vi "Control Panel(WIP).vi"(8 "error in (no error)":errorcluster, 11 "Lockin SR830 in":refnum<class "Lockin SR830.lvclass">) -> (0 "error out":errorcluster, 3 "Lockin SR830 out":refnum<class "Lockin SR830.lvclass">)   [LabVIEW 2017, in "Lockin SR830.lvclass"]
uses:
  Lockin SR830.lvclass
  Lockin SR830.lvclass/Lockin SR830.ctl
  sr830/SR830.lvlib
panel:
  out "?":enum32{"Page 1", "Page 2"}(tab)
  out "Channel 2 Display":dbl
  out "Channel 1 Display":dbl
  out "Ref Freq":dbl[unit]
  in  "Ch 1 Option":T1(ring)
  in  "Ch 2 Option":T2(ring)
  out "Channel 1 display":dbl
  out "Ref freq":dbl[unit]
  in  "Ch 1 option":T1(ring)
  out "Phase":dbl format="%#_13g"
  in  "autophase":bool
  out "External ref":bool=TRUE
  in  "External ref?":bool=TRUE
  in  "Read":bool
  in  "Copy actual to set":bool
  in  "Populate fields with member data":bool
  in  "endprgm":bool
  in  "set":bool
  out "sensdisp":T3(ring) caption="Sensitivity"
  out "tcdisp":T4(ring) caption="Time Const."
  in  "sens":T3(ring) caption="Sensitivity"
  in  "tc":T4(ring) caption="Time Const."
  # "Lock-in Detector Front Panel"
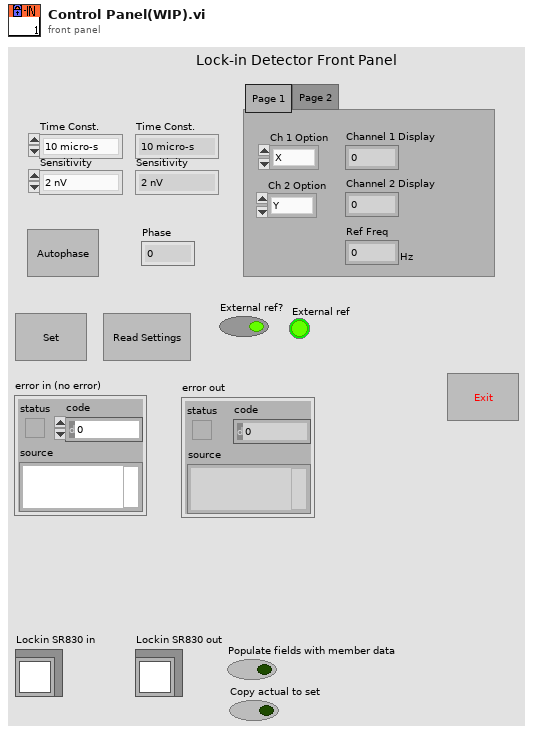
[diagram p1: front panel]
types:
  T1 = enum16{"X", "R", "X Noise", "Aux in 1", "Aux in 2"}
  T2 = enum16{"Y", "Theta", "Y Noise", "Aux in 3", "Aux in 4"}
  T3 = enum16{"2 nV", "5 nV", "10 nV", "20 nV", "50 nV", "100 nV", "200 nV", "500 nV", "1 microV", "2 microV", "5 microV", "10 microV", "20 microV", "50  microV", "100  microV", "200  microV", "500  microV", "1 mV", "2 mV", "5 mV", "10 mV", "20 mV", "50 mV", "100 mV", "200  mV", "500 mV", "1 V"}
  T4 = enum16{"10 micro-s", "30 micro-s", "100 micro-s", "300 micro-s", "1 ms", "3 ms", "10 ms", "30 ms", "100 ms", "300 ms", "1 s", "3 s", "10 s", "30 s", "100 s", "300 s", "1000 s", "30000 s", "10 ks", "30 ks"}
  T5 = typedef "Lockin SR830.lvclass/Sensitivity.ctl" = u16
  T6 = typedef "SR830.lvlib/Tau.ctl" = u16
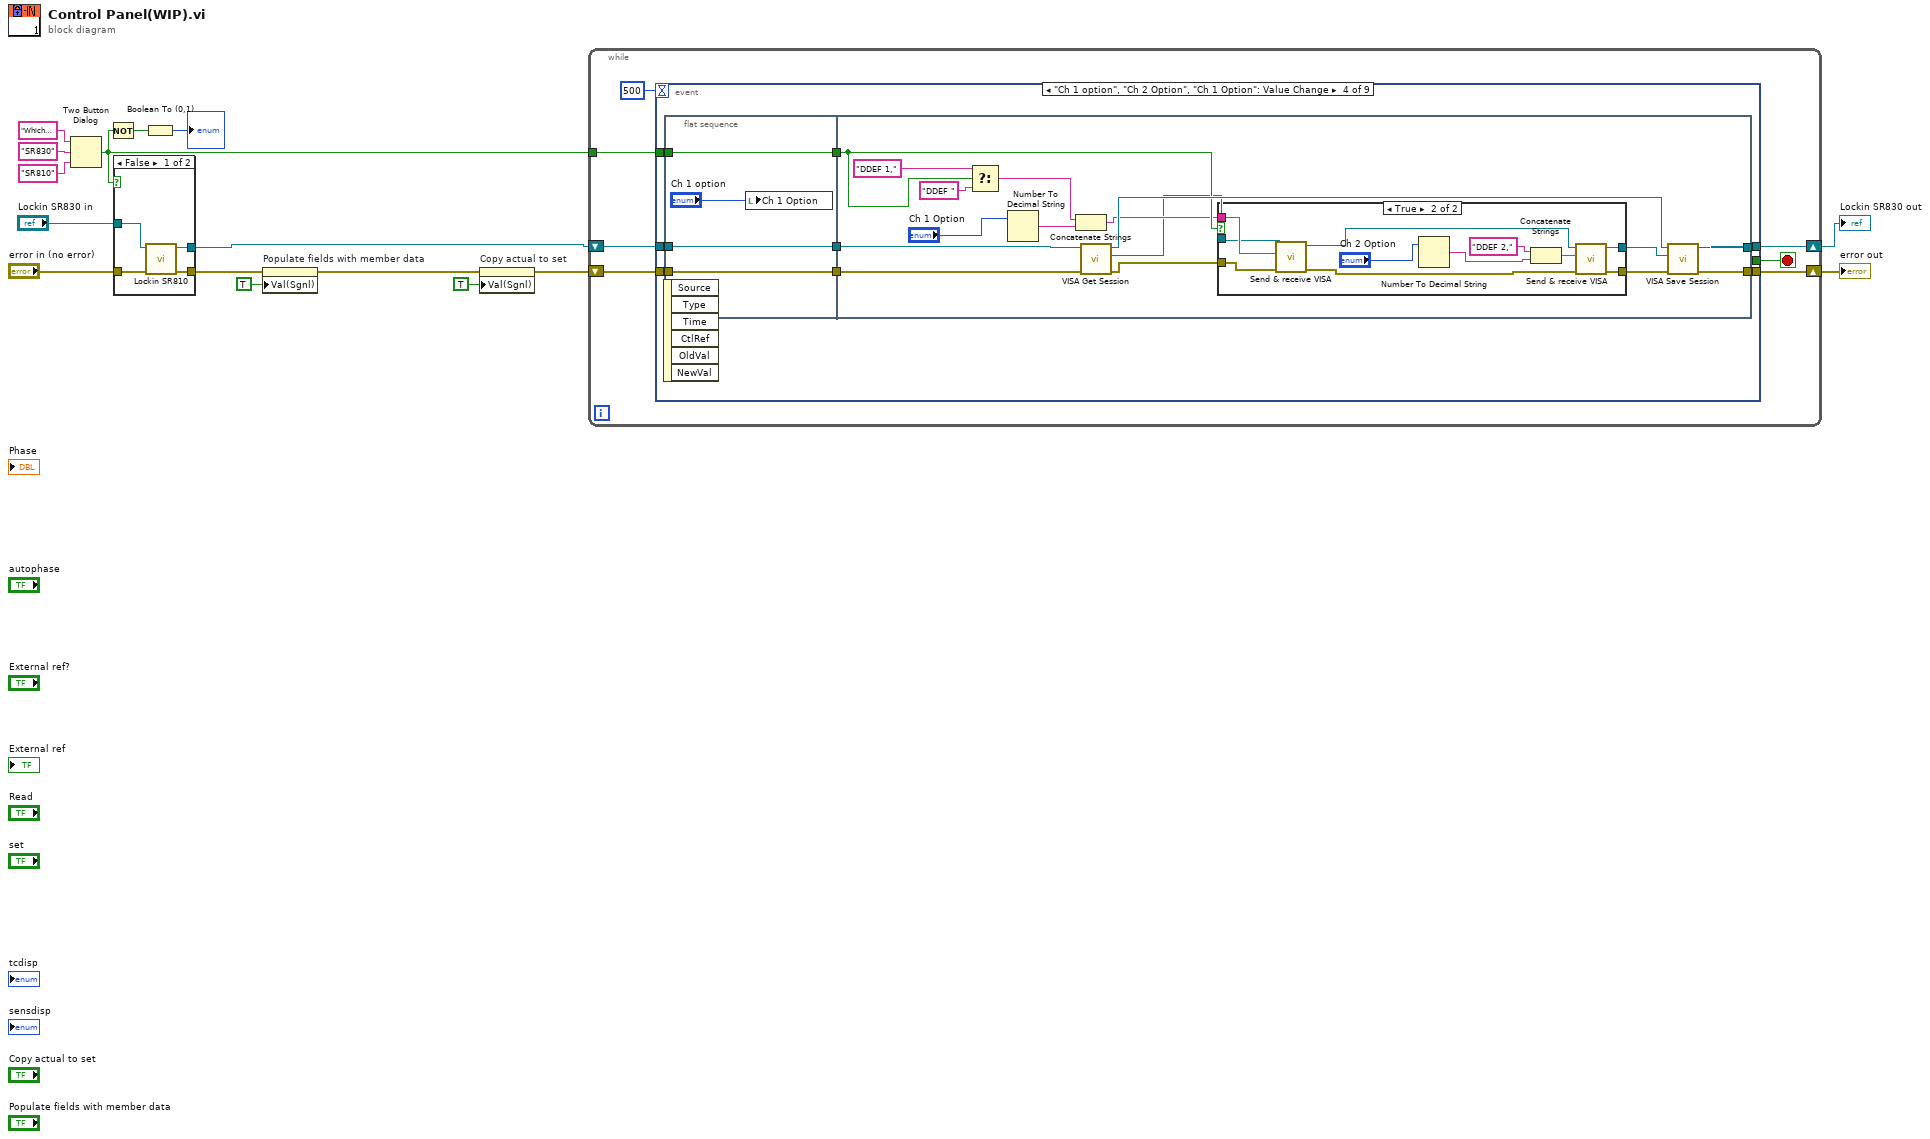
[diagram p0: block diagram]
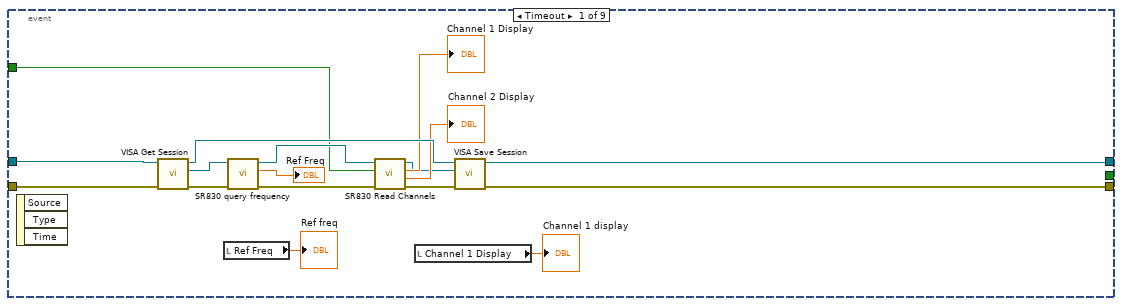
[diagram p2: hidden frame]
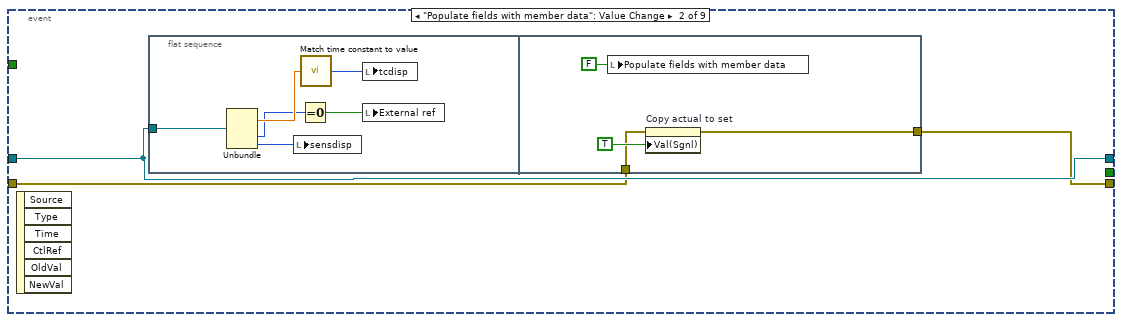
[diagram p3: hidden frame]
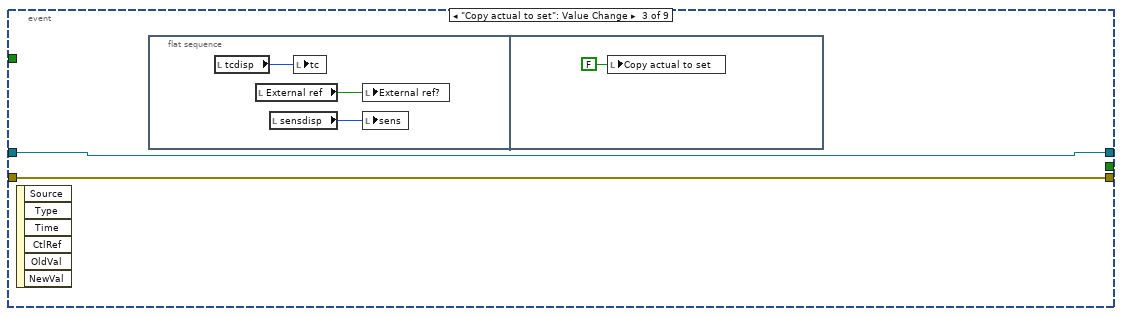
[diagram p4: hidden frame]
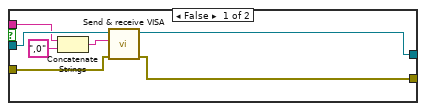
[diagram p5: hidden frame]
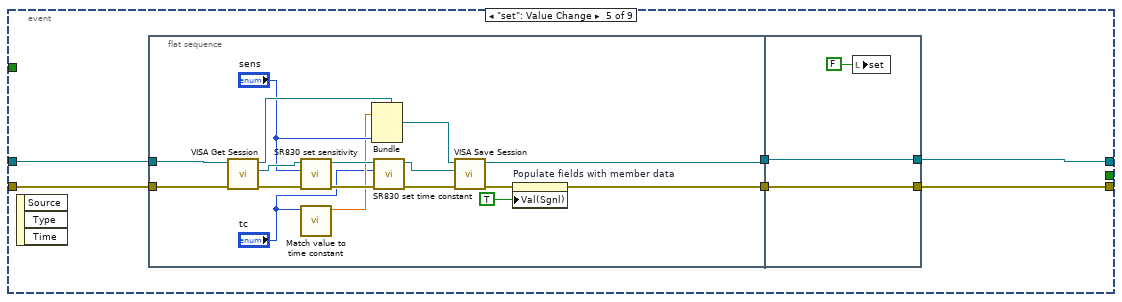
[diagram p6: hidden frame]
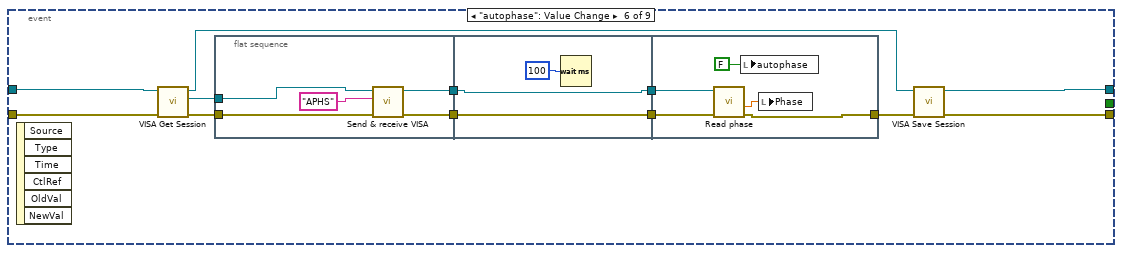
[diagram p7: hidden frame]
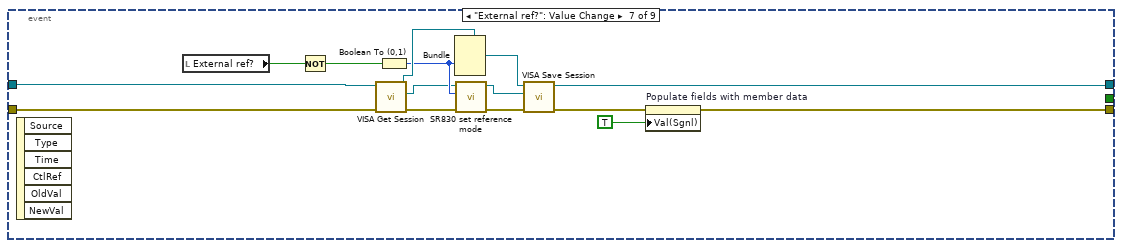
[diagram p8: hidden frame]
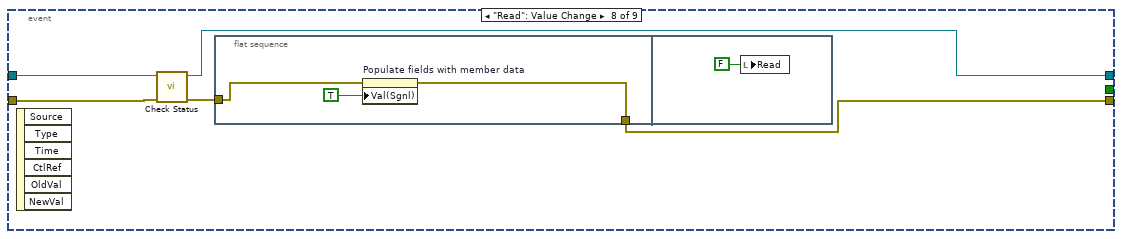
[diagram p9: hidden frame]
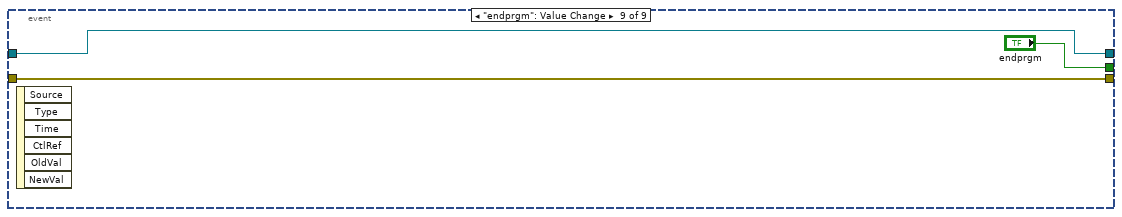
[diagram p10: hidden frame]
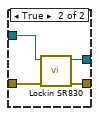
[diagram p11: hidden frame]
diagram:
  n1 = Two Button Dialog(message="Which model Lock-In are you using?", 1:"SR810" ("F button name (\"Cancel\")"), 2:"SR830" ("T button name (\"OK\")")) -> (T button?=w1:bool)
  n2 = Not(x=w1) -> (.not. x?=w3:bool)
  n3 = case shown="False" w1 {
    tunnel: "Lockin SR830 in" -> [w20 w24]
    tunnel: "error in (no error)" -> [w18 w23]
    tunnel: [w17 w22] -> w8
    tunnel: [w19 w21] -> w13
    frame False {
      n4 = call "Lockin SR810.vi"("error in (no error)"=w18, "Lockin SR830 in"=w20) -> ("error out"=w17:errorcluster, "Lockin SR830 out"=w19:refnum<class "Lockin SR830.lvclass">)  [unwired: 8 in]
    }
    frame True {
      n5 = call "Lockin SR830.vi"("error in (no error)"=w23, "Lockin SR830 in"=w24) -> ("error out"=w22:errorcluster, "Lockin SR830 out"=w21:refnum<class "Lockin SR830.lvclass">)  [unwired: 8 in]
    }
  }
  n6 = Boolean To (0,1)(Boolean=w3) -> (0, 1=→"?":i16)
  n7 = property on="Populate fields with member data" class="Bool (strict)"(error in=w8, "Val(Sgnl)"=TRUE) -> (error out=w7:errorcluster)  [unwired: 1 in, 1 out]
  n8 = property on="Copy actual to set" class="Bool (strict)"(error in=w7, "Val(Sgnl)"=TRUE) -> (error out=w6:errorcluster)  [unwired: 1 in, 1 out]
  n9 = while {
    shift-right: [w27] -> w14
    shift-left: w13 -> [w28]
    shift-right: [w29] -> w9
    shift-left: w6 -> [w30]
    tunnel: w1 -> [w25]
    stop <- w31 stop-if-true
    n10 = event shown="[3] \"Ch 1 option\", \"Ch 2 Option\", \"Ch 1 Option\": Value Change" {
      selector: _ -> [_ _ _ _ _ _ _ _ _]
      dyn-events: _ -> [_ _ _ _ _ _ _ _ _]
      timeout: 500 -> [_ _ _ _ _ _ _ _ _]
      tunnel: [_ _ _ _ _ _ _ _ "endprgm"] -> w31
      tunnel: w28 -> [w48 w51 w63 w75 w119 w151 w169 w184 w189]
      tunnel: w30 -> [w44 w50 w62 w74 w118 w148 w167 w183 w190]
      tunnel: [w35 w49 w62 w73 w117 w140 w168 w181 w190] -> w29
      tunnel: [w46 w51 w63 w72 w116 w149 w170 w180 w189] -> w27
      tunnel: w25 -> [w34 _ _ w71 _ _ _ _ _]
      event Timeout {
        n11 = event-data() -> ()  [unwired: 1 in, 3 out]
        n12 = call-dynamic "VISA Get Session.vi"("error in (no error)"=w44, "Instrument.lvclass in"=w48) -> ("error out"=w43:errorcluster, "VISA Resource Name"=w45:refnum<visa-resource-name>, "Instrument.lvclass out"=w47:refnum<class "Lockin SR830.lvclass">)  [unwired: 7 out]
        n13 = local read "Ref Freq"() -> (→"Ref freq":dbl[unit])
        n14 = call "SR830 query frequency.vi"("error in (no error)"=w43, "VISA resource name"=w45) -> ("error out"=w40:errorcluster, "frequency"=→"Ref Freq":dbl[unit], "VISA resource name out"=w41:refnum<visa-resource-name>)  [unwired: 7 in]
        n15 = call "SR830 Read Channels.vi"("error in (no error)"=w40, "830?"=w34, "VISA Resource Name"=w41) -> ("error out"=w36:errorcluster, "output2"=→"Channel 2 Display":dbl, "output1"=→"Channel 1 Display":dbl, "VISA resource name out"=w37:refnum<visa-resource-name>)  [unwired: 5 in]
        n16 = local read "Channel 1 Display"() -> (→"Channel 1 display":dbl)
        n17 = call-dynamic "VISA Save Session.vi"("error in (no error)"=w36, "VISA Resource Name"=w37, "Instrument.lvclass in"=w47) -> ("error out"=w35:errorcluster, "Instrument.lvclass out"=w46:refnum<class "Lockin SR830.lvclass">)  [unwired: 7 out]
      }
      event "Populate fields with member data": Value Change {
        n18 = event-data() -> ()  [unwired: 1 in, 6 out]
        n19 = flat-sequence {
          tunnel: w51 -> [w56]
          tunnel: [w58] -> w49
          tunnel: w50 -> [w59]
          frame #0 {
            n20 = Unbundle(w56) -> (w55:dbl[unit], w52:enum16{"external", "internal"}, w57:T5)  [unwired: 2 out]
            n21 = local write "sensdisp"(w57) -> ()
            n22 = Equal To 0?(x=w52) -> (x = 0?=w53:bool)
            n23 = call "Match time constant to value.vi"("Time constant"=w55) -> ("Tau"=w54:T6)
            n24 = local write "tcdisp"(w54) -> ()
            n25 = local write "External ref"(w53) -> ()
          }
          frame #1 {
            n26 = local write "Populate fields with member data"(FALSE) -> ()
            n27 = property on="Copy actual to set" class="Bool (strict)"(error in=w59, "Val(Sgnl)"=TRUE) -> (error out=w58:errorcluster)  [unwired: 1 in, 1 out]
          }
        }
      }
      event "Copy actual to set": Value Change {
        n28 = event-data() -> ()  [unwired: 1 in, 6 out]
        n29 = flat-sequence {
          frame #0 {
            n30 = local read "tcdisp"() -> (w66:T4)
            n31 = local read "External ref"() -> (w64:bool)
            n32 = local read "sensdisp"() -> (w65:T3)
            n33 = local write "tc"(w66) -> ()
            n34 = local write "External ref?"(w64) -> ()
            n35 = local write "sens"(w65) -> ()
          }
          frame #1 {
            n36 = local write "Copy actual to set"(FALSE) -> ()
          }
        }
      }
      event "Ch 1 option", "Ch 2 Option", "Ch 1 Option": Value Change {
        n37 = event-data() -> ()  [unwired: 1 in, 6 out]
        n38 = flat-sequence {
          tunnel: w71 -> [w77]
          tunnel: w74 -> [w78]
          tunnel: w75 -> [w79]
          tunnel: [w79] -> w70
          tunnel: [w78] -> w69
          tunnel: [w77] -> w68
          tunnel: [w92] -> w73
          tunnel: [w91] -> w72
          tunnel: w70 -> [w95]
          tunnel: w69 -> [w93]
          tunnel: w68 -> [w86]
          frame #0 {
            n39 = local write "Ch 1 Option"("Ch 1 option") -> ()
          }
          frame #1 {
            n40 = Select(t="DDEF 1," ("write buffer"), s=w86, f="DDEF " ("write buffer")) -> (s? t:f=w83:string)
            n41 = Number To Decimal String(number="Ch 1 Option") -> (decimal integer string=w87:string)  [unwired: 1 in]
            n42 = Concatenate Strings(w83, w87) -> (w81:string)
            n43 = call-dynamic "VISA Get Session.vi"("error in (no error)"=w93, "Instrument.lvclass in"=w95) -> ("error out"=w82:errorcluster, "VISA Resource Name"=w80:refnum<visa-resource-name>, "Instrument.lvclass out"=w94:refnum<class "Lockin SR830.lvclass">)  [unwired: 7 out]
            n44 = case shown="True" w86 {
              tunnel: [w96 w113] -> w90
              tunnel: [w97 w112] -> w89
              tunnel: w82 -> [w98 w107]
              tunnel: w81 -> [w101 w106]
              tunnel: w80 -> [w102 w105]
              frame False {
                n45 = Concatenate Strings(w101, ",0" ("string")) -> (w99:string)
                n46 = call "Send & receive VISA.vi"("error in (no error)"=w98, "write buffer"=w99, "VISA resource name"=w102) -> ("error out"=w97:errorcluster, "VISA resource name out"=w96:refnum<visa-resource-name>)  [unwired: 5 in, 2 out]
              }
              frame True {
                n47 = call "Send & receive VISA.vi"("error in (no error)"=w107, "write buffer"=w106, "VISA resource name"=w105) -> ("error out"=w104:errorcluster, "VISA resource name out"=w103:refnum<visa-resource-name>)  [unwired: 5 in, 2 out]
                n48 = Number To Decimal String(number="Ch 2 Option") -> (decimal integer string=w111:string)  [unwired: 1 in]
                n49 = Concatenate Strings("DDEF 2," ("write buffer"), w111) -> (w109:string)
                n50 = call "Send & receive VISA.vi"("error in (no error)"=w104, "write buffer"=w109, "VISA resource name"=w103) -> ("error out"=w112:errorcluster, "VISA resource name out"=w113:refnum<visa-resource-name>)  [unwired: 5 in, 2 out]
              }
            }
            n51 = call-dynamic "VISA Save Session.vi"("error in (no error)"=w89, "VISA Resource Name"=w90, "Instrument.lvclass in"=w94) -> ("error out"=w92:errorcluster, "Instrument.lvclass out"=w91:refnum<class "Lockin SR830.lvclass">)  [unwired: 7 out]
          }
        }
      }
      event "set": Value Change {
        n52 = event-data() -> ()  [unwired: 1 in, 3 out]
        n53 = flat-sequence {
          tunnel: w119 -> [w136]
          tunnel: w118 -> [w134]
          tunnel: [w127] -> w115
          tunnel: [w130] -> w114
          tunnel: [w138] -> w116
          tunnel: [w139] -> w117
          tunnel: w115 -> [w139]
          tunnel: w114 -> [w138]
          frame #0 {
            n54 = call-dynamic "VISA Get Session.vi"("error in (no error)"=w134, "Instrument.lvclass in"=w136) -> ("error out"=w133:errorcluster, "VISA Resource Name"=w135:refnum<visa-resource-name>, "Instrument.lvclass out"=w126:refnum<class "Lockin SR830.lvclass">)  [unwired: 7 out]
            n55 = call "SR830 set sensitivity.vi"("error in (no error)"=w133, "Sensitivity"="sens", "VISA resource name"=w135) -> ("error out"=w131:errorcluster, "VISA resource name out"=w132:refnum<visa-resource-name>)  [unwired: 7 in]
            n56 = call "Match value to time constant.vi"("Tau"="tc") -> ("time constant"=w123:dbl[unit])  [unwired: 10 in]
            n57 = Bundle(cluster=w126, w123, "sens") -> (w124:refnum<class "Lockin SR830.lvclass">)  [unwired: 3 in]
            n58 = call "SR830 set time constant.vi"("error in (no error)"=w131, "Tau"="tc", "VISA resource name"=w132) -> ("error out"=w121:errorcluster, "VISA resource name out"=w120:refnum<visa-resource-name>)  [unwired: 7 in]
            n59 = call-dynamic "VISA Save Session.vi"("error in (no error)"=w121, "VISA Resource Name"=w120, "Instrument.lvclass in"=w124) -> ("error out"=w128:errorcluster, "Instrument.lvclass out"=w130:refnum<class "Lockin SR830.lvclass">)  [unwired: 7 out]
            n60 = property on="Populate fields with member data" class="Bool (strict)"(error in=w128, "Val(Sgnl)"=TRUE) -> (error out=w127:errorcluster)  [unwired: 1 in, 1 out]
          }
          frame #1 {
            n61 = local write "set"(FALSE) -> ()
          }
        }
      }
      event "autophase": Value Change {
        n62 = event-data() -> ()  [unwired: 1 in, 6 out]
        n63 = call-dynamic "VISA Get Session.vi"("error in (no error)"=w148, "Instrument.lvclass in"=w151) -> ("error out"=w146:errorcluster, "VISA Resource Name"=w147:refnum<visa-resource-name>, "Instrument.lvclass out"=w150:refnum<class "Lockin SR830.lvclass">)  [unwired: 7 out]
        n64 = flat-sequence {
          tunnel: w147 -> [w156]
          tunnel: w146 -> [w155]
          tunnel: [w153] -> w144
          tunnel: [w152] -> w142
          tunnel: [w158] -> w145
          tunnel: w144 -> [w158]
          tunnel: [w157] -> w143
          tunnel: w142 -> [w157]
          tunnel: w145 -> [w164]
          tunnel: w143 -> [w163]
          tunnel: [w161] -> w141
          frame #0 {
            n65 = call "Send & receive VISA.vi"("error in (no error)"=w155, "write buffer"="APHS", "VISA resource name"=w156) -> ("error out"=w152:errorcluster, "VISA resource name out"=w153:refnum<visa-resource-name>)  [unwired: 5 in, 2 out]
          }
          frame #1 {
            n66 = Wait (ms)(milliseconds to wait=u32 100) -> ()  [unwired: 1 out]
          }
          frame #2 {
            n67 = call "Read phase.vi"("error in (no error)"=w163, "VISA resource name"=w164) -> ("error out"=w161:errorcluster, "phase"=w162:dbl)  [unwired: 7 in, 1 out]
            n68 = local write "autophase"(FALSE) -> ()
            n69 = local write "Phase"(w162) -> ()
          }
        }
        n70 = call-dynamic "VISA Save Session.vi"("error in (no error)"=w141, "Instrument.lvclass in"=w150) -> ("error out"=w140:errorcluster, "Instrument.lvclass out"=w149:refnum<class "Lockin SR830.lvclass">)  [unwired: 1 in, 7 out]
      }
      event "External ref?": Value Change {
        n71 = event-data() -> ()  [unwired: 1 in, 6 out]
        n72 = local read "External ref?"() -> (w172:bool)
        n73 = Not(x=w172) -> (.not. x?=w173:bool)
        n74 = call-dynamic "VISA Get Session.vi"("error in (no error)"=w167, "Instrument.lvclass in"=w169) -> ("error out"=w166:errorcluster, "VISA Resource Name"=w165:refnum<visa-resource-name>, "Instrument.lvclass out"=w177:refnum<class "Lockin SR830.lvclass">)  [unwired: 7 out]
        n75 = Boolean To (0,1)(Boolean=w173) -> (0, 1=w171:i16)
        n76 = Bundle(cluster=w177, w171) -> (w176:refnum<class "Lockin SR830.lvclass">)  [unwired: 4 in]
        n77 = call "SR830 set reference mode.vi"("error in (no error)"=w166, "reference mode"=w171, "VISA resource name"=w165) -> ("error out"=w175:errorcluster, "VISA resource name out"=w174:refnum<visa-resource-name>)  [unwired: 7 in]
        n78 = call-dynamic "VISA Save Session.vi"("error in (no error)"=w175, "VISA Resource Name"=w174, "Instrument.lvclass in"=w176) -> ("error out"=w178:errorcluster, "Instrument.lvclass out"=w170:refnum<class "Lockin SR830.lvclass">)  [unwired: 7 out]
        n79 = property on="Populate fields with member data" class="Bool (strict)"(error in=w178, "Val(Sgnl)"=TRUE) -> (error out=w168:errorcluster)  [unwired: 1 in, 1 out]
      }
      event "Read": Value Change {
        n80 = event-data() -> ()  [unwired: 1 in, 6 out]
        n81 = call-dynamic "Check Status.vi"("error in (no error)"=w183, "Lockin SR830 in"=w184) -> ("error out"=w182:errorcluster, "Lockin SR830 out"=w180:refnum<class "Lockin SR830.lvclass">)  [unwired: 6 in, 2 out]
        n82 = flat-sequence {
          tunnel: w182 -> [w186]
          tunnel: [w185] -> w181
          frame #0 {
            n83 = property on="Populate fields with member data" class="Bool (strict)"(error in=w186, "Val(Sgnl)"=TRUE) -> (error out=w185:errorcluster)  [unwired: 1 in, 1 out]
          }
          frame #1 {
            n84 = local write "Read"(FALSE) -> ()
          }
        }
      }
      event "endprgm": Value Change {
        n85 = event-data() -> ()  [unwired: 1 in, 6 out]
      }
    }
  }
  "error out" <- w9
  "Lockin SR830 out" <- w14
